vi "PH_SRDG645.show Device Errors.vi"(1 "Device Errors":cluster{"code":i32, "Text":string}[](array[cluster]), 2 "error in":errorcluster, 3 "Ref Device Errors":refnum<vi>) -> (0 "error out":errorcluster)   [LabVIEW 2014, in "PH_SRDG645.lvlib"]
doc: "This VI shows the Device Errors at the panel."
uses:
  PH_SRDG645.lvlib
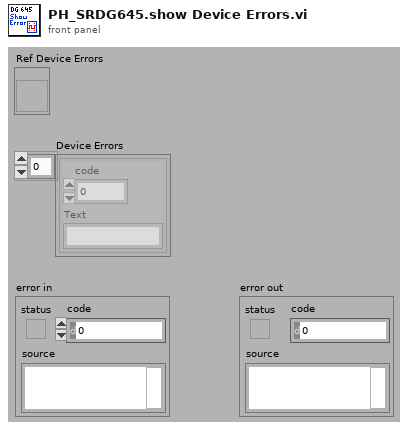
[diagram p1: front panel]
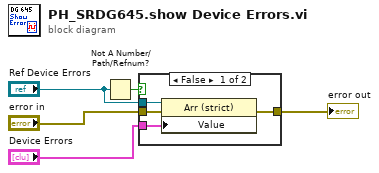
[diagram p0: block diagram]
diagram:
  n1 = Not A Number/Path/Refnum?(number/path/refnum="Ref Device Errors") -> (NaN/Path/Refnum?=w1:bool)
  n2 = case shown="False" w1 {
    tunnel: "error in" -> [w9 w10]
    tunnel: [w8 w10] -> w3
    tunnel: "Ref Device Errors" -> [w7 _]
    tunnel: "Device Errors" -> [w6 _]
    frame False {
      n3 = property class="Arr (strict)"(reference=w7, error in=w9, "Value"=w6) -> (error out=w8:errorcluster)  [unwired: 1 out]
    }
    frame True {
    }
  }
  "error out" <- w3
